vi "Acel_calib_calib.vi"(0 "Acel Cal measurements in":sgl[][](array[numeric]), 7 "Frecuencia\nmuestreo":dbl, 9 "Pattern frequency (Hz)":dbl, 11 "Pattern\namplitude":dbl) -> (4 "Acel Cal measurements out":dbl[][](array[numeric]), 6 "Calibration parameter":dbl, 8 "Sensivity (mV/g)":dbl, 10 "Reporting 4":string, 15 "Calibration OK":bool)   [LabVIEW 2015]
uses:
  <vilib>/measure/NI_MAPro.lvlib
  <vilib>/measure/madcrms.llb/Basic Averaged DC-RMS for 1 Chan.vi
  <vilib>/Analysis/NI_AALPro.lvlib
  <vilib>/Analysis/5stat.llb/RMS (DBL).vi
  <vilib>/Analysis/NI_AALBase.lvlib
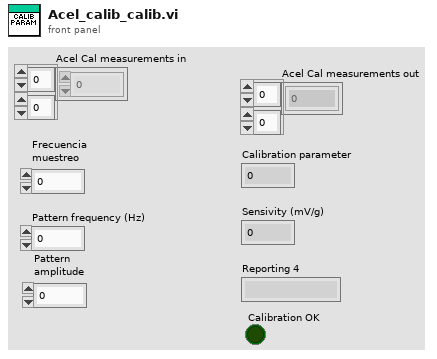
[diagram p1: front panel]
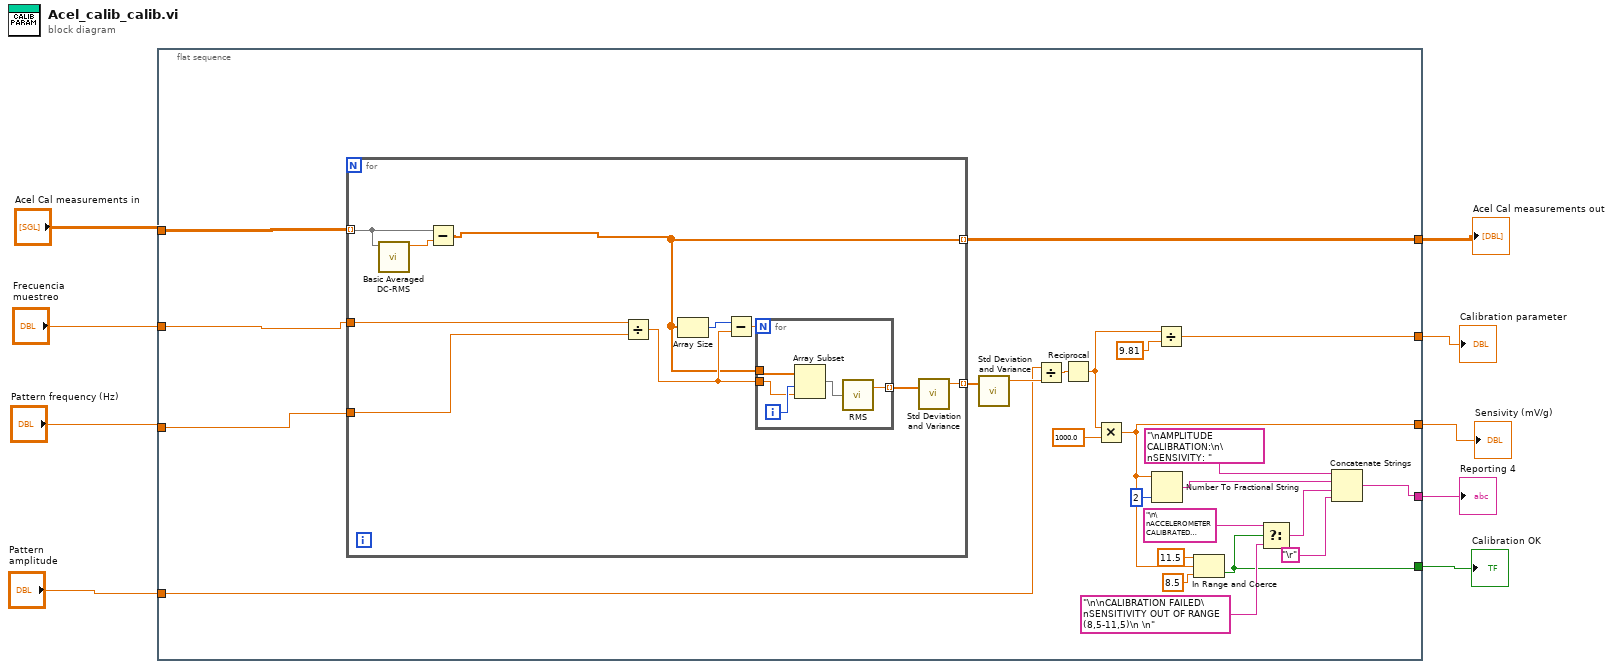
[diagram p0: block diagram]
diagram:
  n1 = flat-sequence {
    tunnel: "Acel Cal measurements in" -> [w28]
    tunnel: [w27] -> w2
    tunnel: "Frecuencia\nmuestreo" -> [w25]
    tunnel: "Pattern frequency (Hz)" -> [w24]
    tunnel: "Pattern\namplitude" -> [w23]
    tunnel: [w22] -> w7
    tunnel: [w19] -> w6
    tunnel: [w13] -> w8
    tunnel: [w12] -> w9
    frame #0 {
      n2 = for {
        tunnel: w28 -> [w42] mode=indexing
        tunnel: w25 -> [w38]
        tunnel: w24 -> [w35]
        tunnel: [w36] -> w33 mode=indexing
        tunnel: [w34] -> w27 mode=indexing
        n3 = call-poly <vilib>:"Basic Averaged DC-RMS.vi"("signal in"=w42) -> ("DC value"=w43:dbl)  [unwired: 7 in, 3 out]
        n4 = Subtract(x=w42, y=w43) -> (x-y=w34:dbl[])
        n5 = Divide(x=w38, y=w35) -> (x/y=w39:dbl)
        n6 = Array Size(array=w34) -> (size(s)=w40:i32)
        n7 = Subtract(x=w40, y=w39) -> (x-y=w41:dbl)
        n8 = for {
          N: w41 -> [_]
          tunnel: w39 -> [w45]
          tunnel: [w48] -> w37 mode=indexing
          tunnel: w34 -> [w47]
          i -> [w46]
          n9 = Array Subset(array=w47, index=w46, length=w45) -> (w44:dbl[])
          n10 = call-poly <vilib>:"RMS.vi"("X"=w44) -> ("rms value"=w48:dbl)  [unwired: 1 out]
        }
        n11 = call <vilib>:"Std Deviation and Variance.vi"("X"=w37) -> ("mean"=w36:dbl)  [unwired: 1 in, 2 out]
      }
      n12 = call <vilib>:"Std Deviation and Variance.vi"("X"=w33) -> ("mean"=w32:dbl)  [unwired: 1 in, 2 out]
      n13 = Divide(x=w23, y=w32) -> (x/y=w30:dbl)
      n14 = Reciprocal(x=w30) -> (1/x=w26:dbl)
      n15 = Multiply(x=w26, y=1000.0) -> (x*y=w19:dbl)
      n16 = Number To Fractional String(number=w19, precision (6)=i16 2) -> (F-format string=w15:string)  [unwired: 2 in]
      n17 = Divide(x=w26, y=9.81) -> (x/y=w22:dbl)
      n18 = In Range and Coerce(upper limit=11.5, x=w19, lower limit=8.5) -> (In Range?=w13:bool)  [unwired: 1 out]
      n19 = Select(t="\n\nACCELEROMETER CALIBRATED CORRECTLY\n \n", s=w13, f="\n\nCALIBRATION FAILED\nSENSITIVITY OUT OF RANGE (8,5-11,5)\n \n") -> (s? t:f=w14:string)
      n20 = Concatenate Strings("\nAMPLITUDE CALIBRATION:\n\nSENSIVITY: ", w15, w14, "\r") -> (w12:string)
    }
  }
  "Reporting 4" <- w9
  "Calibration OK" <- w8
  "Calibration parameter" <- w7
  "Sensivity (mV/g)" <- w6
  "Acel Cal measurements out" <- w2
